vi "Stop Core.vi"(10 "final error code":i32, 11 "Nested in":refnum<class "UI VISA Terminal.lvclass">) -> (3 "Nested out":refnum<class "UI VISA Terminal.lvclass">)   [LabVIEW 2025, in "UI VISA Terminal.lvlib" / "UI VISA Terminal.lvclass"]
doc: "(<B>Filename</B>: Actor Framework.lvlib:Actor.lvclass:Stop Core.vi)\n\nDefines what the actor does before it stops. Use the <B>final error code</B> input to determine whether the actor shut down in response to an error.\n\nBy default, this method does nothing. A descendant class may override it to define behavior, such as shutting down any processes the actor initiated in its override of the Actor Core method."
uses:
  UI VISA Terminal.lvclass
  <vilib>/ActorFramework/Actor/Actor.lvclass
  UI VISA Terminal.lvclass/UI VISA Terminal.ctl
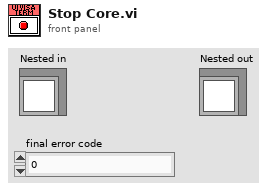
[diagram p1: front panel]
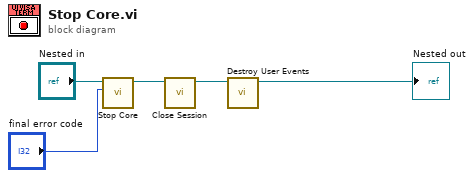
[diagram p0: block diagram]
diagram:
  n1 = call-parent "Stop Core.vi"("final error code"="final error code", "Actor in"="Nested in") -> ("Actor out"=w3:refnum<class "UI VISA Terminal.lvclass">)  [unwired: 9 in]
  n2 = call-dynamic "Close Session.vi"("UI VISA Terminal in"=w3) -> ("UI VISA Terminal out"=w1:refnum<class "UI VISA Terminal.lvclass">)  [unwired: 9 in, 1 out]
  n3 = call "Destroy User Events.vi"("UI Template in"=w1) -> ("UI Template out"=→"Nested out":refnum<class "UI VISA Terminal.lvclass">)  [unwired: 10 in]
